vi "Filter_String_Parser.vi"(8 "error in":errorcluster, 11 "Filter String":string="Protocol == UDP AND Length > 0.7 OR Source == 192.168.1.1") -> (0 "error constant":errorcluster, 1 "Comparators":T1(array[cluster]), 3 "Boolean Connectors":string[](array[string]))   [LabVIEW 2025, in "Table_Filtering.lvlib"]
uses:
  Table_Filtering.lvlib
  <vilib>/Utility/error.llb/whitespace.ctl
  <vilib>/Utility/error.llb/Trim Whitespace One-Sided.vi
  <vilib>/regexp/Match Regular Expression.xnode
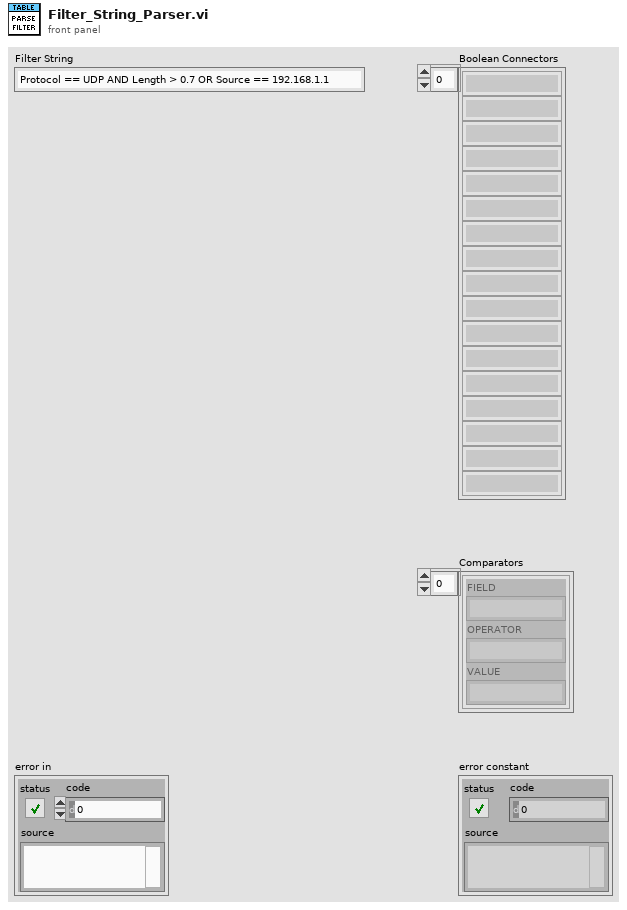
[diagram p1: front panel]
types:
  T1 = cluster{"FIELD":string, "OPERATOR":string, "VALUE":string}[]
  T2 = typedef "whitespace.ctl" = u16
  T3 = cluster{"FIELD":string, "OPERATOR":string, "VALUE":string}
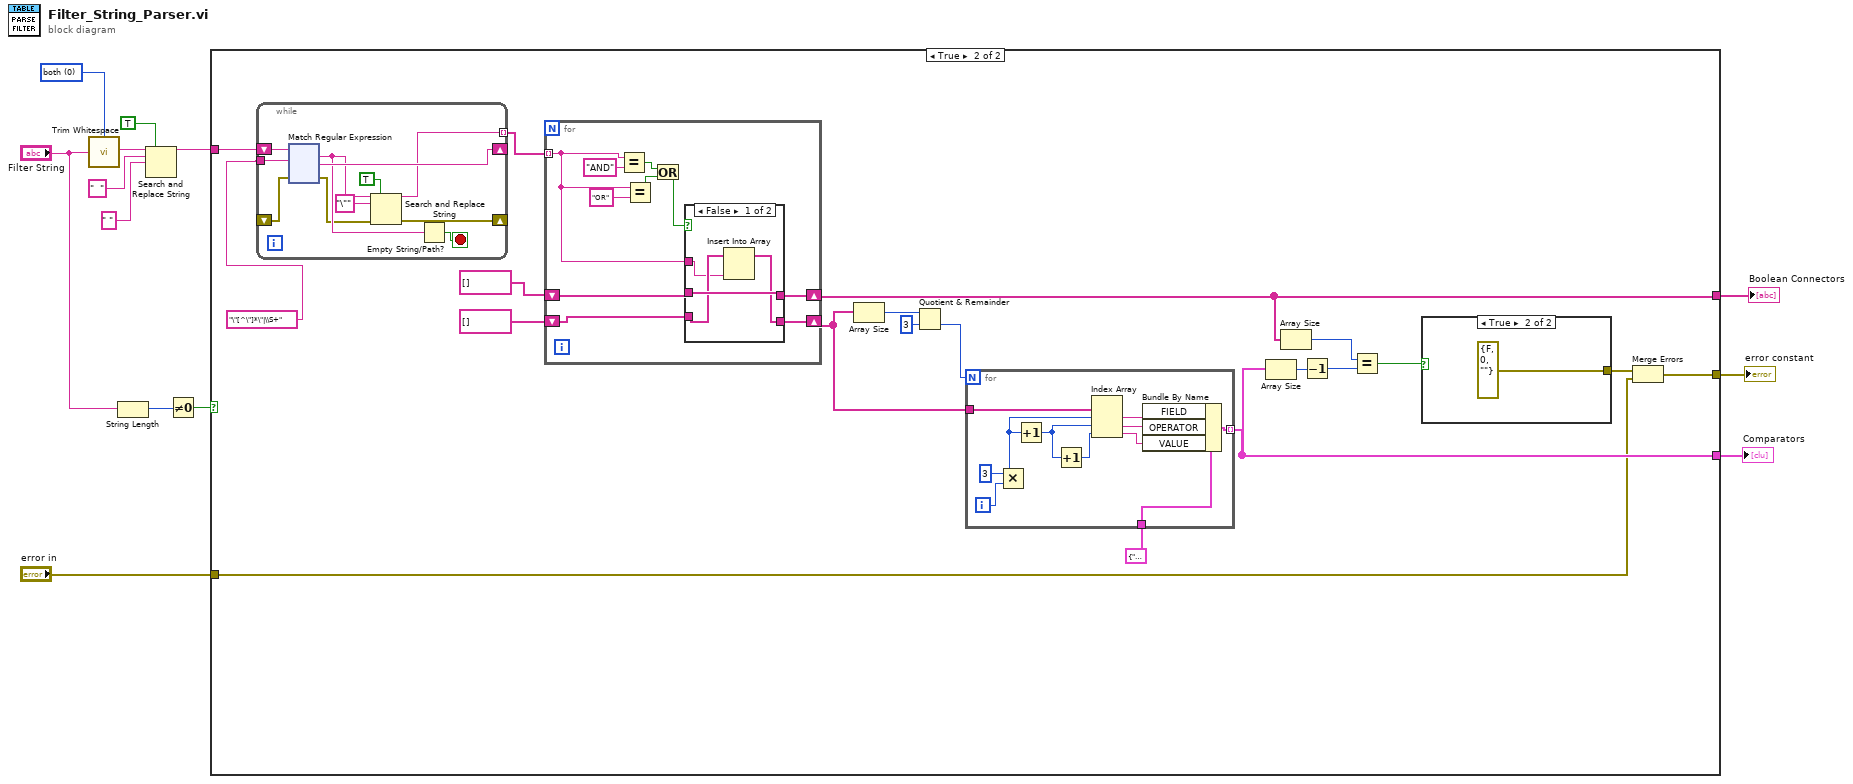
[diagram p0: block diagram]
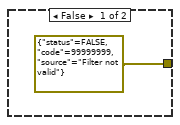
[diagram p3: hidden frame]
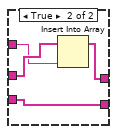
[diagram p4: hidden frame]
diagram:
  w6 = T2 0 items=["both", "start of string", "end of string"] ("location (both)")
  n1 = call <vilib>:"Trim Whitespace.vi"("string"="Filter String", "location (both)"=w6) -> ("trimmed string"=w4:string)
  n2 = String Length(string="Filter String") -> (length=w13:i32)
  n3 = Search and Replace String(replace all?=TRUE ("replace all? (F)"), input string=w4, search string="  ", replace string=" " ("replace string (\"\")")) -> (result string=w5:string)  [unwired: 4 in, 3 out]
  n4 = Not Equal To 0?(x=w13) -> (x != 0?=w12:bool)
  n5 = case shown="True" w12 {
    tunnel: w5 -> [_ w16]
    tunnel: [_ w26] -> w11
    tunnel: [_ w23] -> w10
    tunnel: [w14 w20] -> w9
    tunnel: "error in" -> [w14 w18]
    frame False {
    }
    frame True {
      n6 = while {
        tunnel: "\"[^\"]*\"|\\S+" ("regular expression") -> [w43]
        shift-right: [w41] -> _
        shift-left: w16 -> [w44]
        tunnel: [w34] -> w17 mode=indexing
        shift-right: [w36] -> _
        shift-left: _ -> [w35]
        stop <- w42 stop-if-true
        n7 = xnode "Match Regular Expression"("input string"=w44, "regular expression"=w43, "error in"=w35) -> ("whole match"=w40:string, "after match"=w41:string, "error out"=w37:errorcluster)  [unwired: 3 in, 2 out]
        n8 = Search and Replace String(replace all?=TRUE ("replace all? (F)"), input string=w40, search string="\"", error in=w37) -> (result string=w34:string, error out=w36:errorcluster)  [unwired: 4 in, 2 out]
        n9 = Empty String/Path?(string/path=w40) -> (empty?=w42:bool)
      }
      n10 = for {
        tunnel: w17 -> [w179] mode=indexing
        shift-right: [w175] -> w23
        shift-left: string[] [] -> [w178]
        shift-right: [w176] -> w29
        shift-left: string[] [] -> [w177]
        n11 = Equal?(x=w179, y="AND") -> (x = y?=w184:bool)
        n12 = Equal?(x=w179, y="OR") -> (x = y?=w181:bool)
        n13 = Or(x=w184, y=w181) -> (x .or. y?=w180:bool)
        n14 = case shown="False" w180 {
          tunnel: w179 -> [w186 w190]
          tunnel: w178 -> [w188 w191]
          tunnel: [w188 w189] -> w175
          tunnel: w177 -> [w187 w192]
          tunnel: [w185 w192] -> w176
          frame False {
            n15 = Insert Into Array(array=w187, new element=w186) -> (w185:string[])  [unwired: 1 in]
          }
          frame True {
            n16 = Insert Into Array(array=w191, new element=w190) -> (w189:string[])  [unwired: 1 in]
          }
        }
      }
      n17 = Array Size(array=w29) -> (size(s)=w32:i32)
      n18 = Quotient & Remainder(x=w32, y=3) -> (floor(x/y)=w27:i32)  [unwired: 1 out]
      n19 = for {
        N: w27 -> [_]
        tunnel: w29 -> [w174]
        tunnel: T3 {"FIELD"="", "OPERATOR"="", "VALUE"=""} -> [w168]
        tunnel: [w164] -> w26 mode=indexing
        i -> [w173]
        n20 = Multiply(x=3, y=w173) -> (x*y=w171:i32)
        n21 = Increment(x=w171) -> (x+1=w169:i32)
        n22 = Increment(x=w169) -> (x+1=w170:i32)
        n23 = Index Array(array=w174, index #1=w171, index #2=w169, index #3=w170) -> (element #1=w167:string, element #2=w166:string, element #3=w165:string)
        n24 = Bundle By Name(cluster=w168, "FIELD"=w167, "OPERATOR"=w166, "VALUE"=w165) -> (w164:T3)
      }
      n25 = Array Size(array=w26) -> (size(s)=w24:i32)
      n26 = Array Size(array=w23) -> (size(s)=w25:i32)
      n27 = Decrement(x=w24) -> (x-1=w22:i32)
      n28 = Equal?(x=w25, y=w22) -> (x = y?=w21:bool)
      n29 = case shown="True" w21 {
        tunnel: [errorcluster {"status"=FALSE, "code"=99999999, "source"="Filter not valid"} ("error constant") errorcluster {"status"=FALSE, "code"=0, "source"=""} ("error constant")] -> w19
        frame False {
        }
        frame True {
        }
      }
      n30 = Merge Errors(w19, w18) -> (w20:errorcluster)
    }
  }
  "Boolean Connectors" <- w10
  "Comparators" <- w11
  "error constant" <- w9
